vi "临界安全监督数据处理.vi"() -> ()   [LabVIEW 2020]
uses:
  <vilib>/Utility/miscctls.llb/LVAnnotationListTypeDef.ctl
  <vilib>/Analysis/6fits.llb/Curve Fitting Criteria.ctl
  <vilib>/Utility/miscctls.llb/LVRowAndColumnTypeDef.ctl
  <vilib>/Utility/inputDevices.llb/mouseAcquire.vi
  <vilib>/Analysis/NI_AALPro.lvlib
panel:
  in  "背景色":bool
  in  "临界途径选择":u16(ring)
  in  "表象周期标尺\n   手动调整":bool
  in  "Min+":bool
  in  "Min-":bool
  in  "Max+":bool
  in  "Max-":bool
  out "左选标时刻":timestamp
  out "总时长":dbl
  in  "保存表格":bool
  in  "添加记录":bool
  out "Table":string[][](table) caption="表格"
  out "Axis Info":T1 caption="轴信息"
  in  "曲线标尺":bool[](array[boolean])
  in  "曲线隐显":bool[](array[boolean])
  out "提示信息":string
  in  "开始计算":bool
  in  "重选文件":bool
  in  "退出程序":bool
  out "filepath":path caption="数据文件路径和名称"
  out "数据采集起止时间":string
  out "中间段数据个数":i32
  out "左选标位置":i32
  out "右选标位置":i32
  out "选段斜率":sgl[](array[numeric])
  out "通量平均值":sgl[](array[numeric])
  out "表象周期平均（秒）":sgl[](array[numeric])
  out "临界途径平均值":sgl[](array[numeric])
  out "【文件波形】":dbl[][](graph)
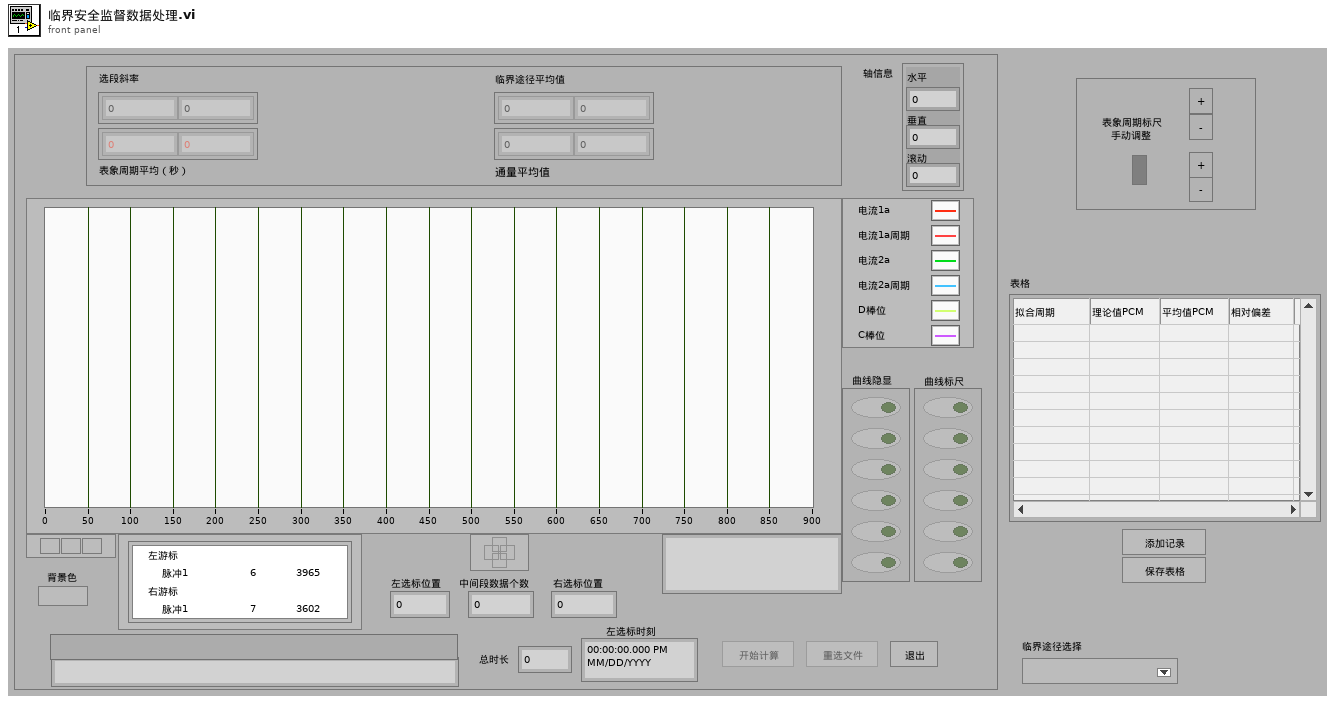
[diagram p1: front panel]
types:
  T1 = cluster{"Horizontal":i32, "Vertical":i32, "Scrolling":i32}
  T2 = enum8{"Enabled", "Disabled", "Disabled and Grayed Out"}
  T3 = typedef "LVAnnotationListTypeDef.ctl" = cluster{"Name":string, "Color":u32, "Style":u8, "Point Style":u8, "Name Visible":bool, "Allow Drag":bool, "Annotation Mode":u32, "Plot":i32, "Index":i32, "Position":cluster{"X":dbl, "Y":dbl}, "X Scale":u32, "Y Scale":u32, "Show Arrow":bool, "Lock Name":bool, "Plot Area":i32, "Label Offset":cluster{"X":dbl, "Y":dbl}}[]
  T4 = cluster{"Name":string, "Color":u32, "Style":u8, "Point Style":u8, "Name Visible":bool, "Allow Drag":bool, "Annotation Mode":u32, "Plot":i32, "Index":i32, "Position":cluster{"X":dbl, "Y":dbl}, "X Scale":u32, "Y Scale":u32, "Show Arrow":bool, "Lock Name":bool, "Plot Area":i32, "Label Offset":cluster{"X":dbl, "Y":dbl}}
  T5 = enum16{"open", "replace", "create", "open or create", "replace or create", "replace or create with confirmation"}
  T6 = typedef "LVRowAndColumnTypeDef.ctl" = cluster{"Row":i32, "Column":i32}
  T7 = cluster{"button 1":bool, "button 2":bool, "button 3":bool, "button 4":bool}
  T8 = typedef "LVCursorListTypeDef.ctl" = cluster{"Name":string, "Color":u32, "Style":u8, "Point Style":u8, "Name Visible":bool, "Allow Drag":bool, "Cursor Mode":u32, "Plot":i32, "Index":i32, "Position":cluster{"X":dbl, "Y":dbl}, "X Scale":u32, "Y Scale":u32, "Watch Plots":i32[], "Watch All Plots":bool, "Plot Area":i32, "Label Offset":cluster{"X":dbl, "Y":dbl}}[]
  T9 = cluster{"Name":string, "Color":u32, "Style":u8, "Point Style":u8, "Name Visible":bool, "Allow Drag":bool, "Cursor Mode":u32, "Plot":i32, "Index":i32, "Position":cluster{"X":dbl, "Y":dbl}, "X Scale":u32, "Y Scale":u32, "Watch Plots":i32[], "Watch All Plots":bool, "Plot Area":i32, "Label Offset":cluster{"X":dbl, "Y":dbl}}
  T10 = typedef "NI_AALPro.lvlib/Curve Fitting Criteria.ctl" = u16
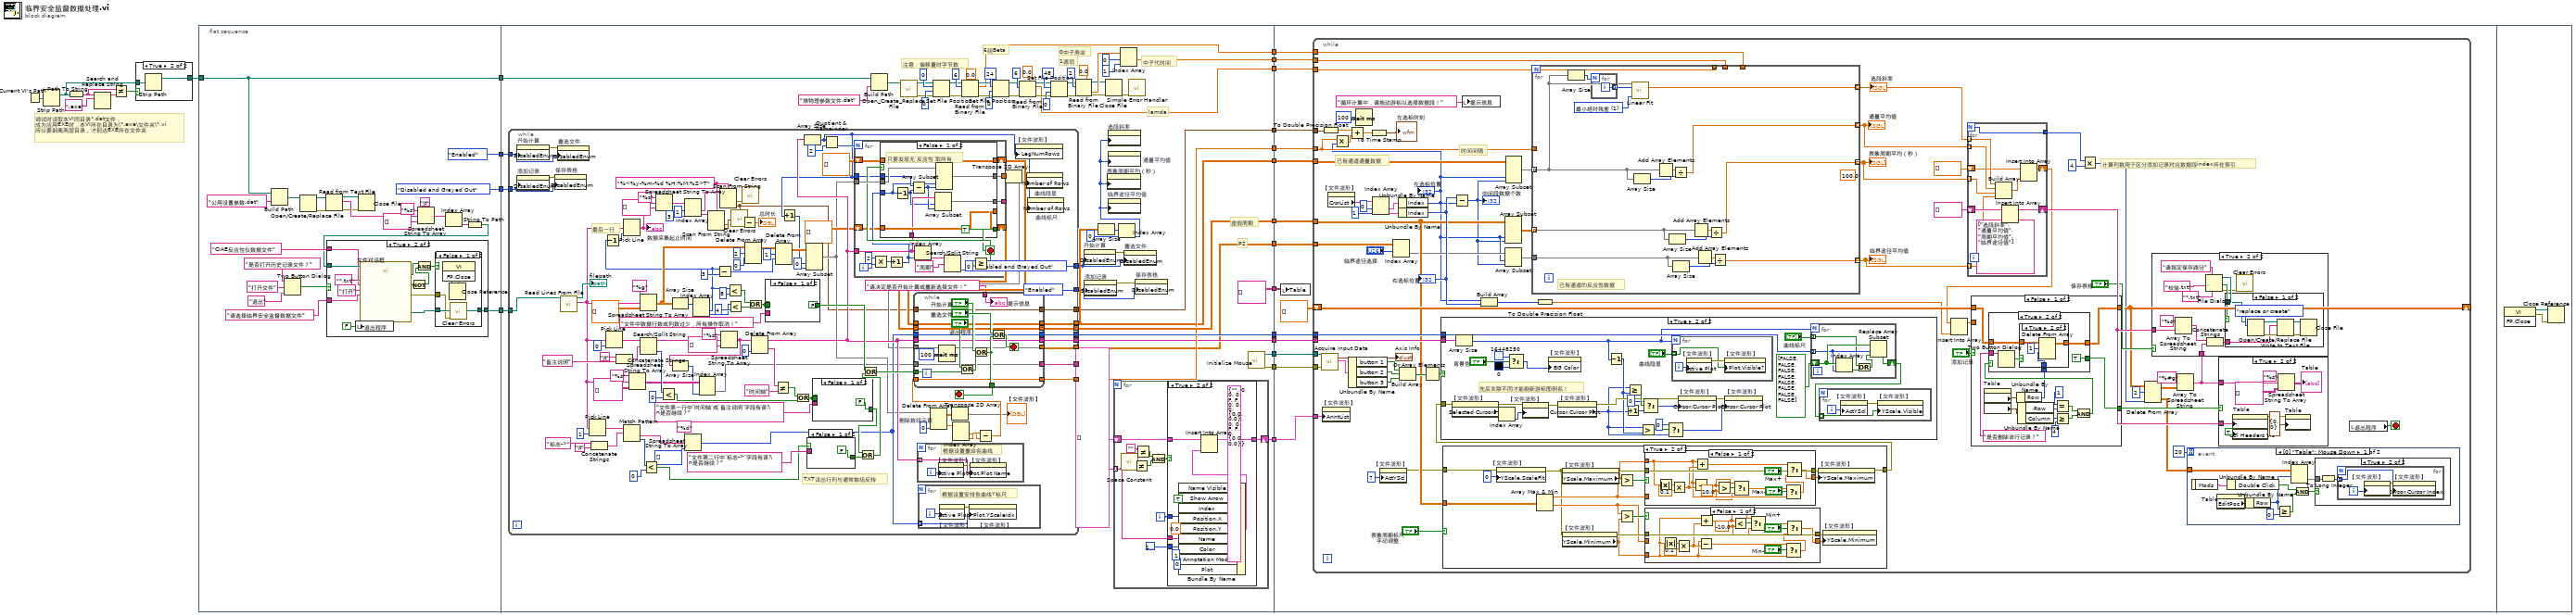
[diagram p0: block diagram]
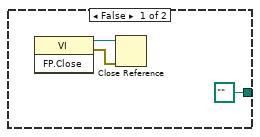
[diagram p3: hidden frame]
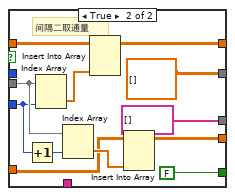
[diagram p6: hidden frame]
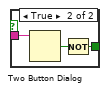
[diagram p7: hidden frame]
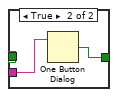
[diagram p8: hidden frame]
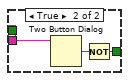
[diagram p9: hidden frame]
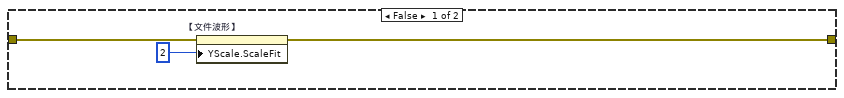
[diagram p10: hidden frame]
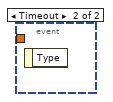
[diagram p14: hidden frame]
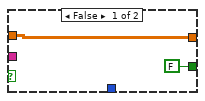
[diagram p18: hidden frame]
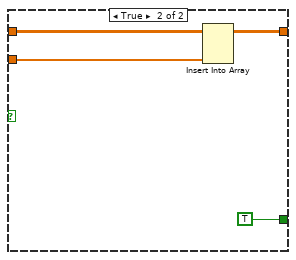
[diagram p20: hidden frame]
diagram:
  # "调试时读取本VI同目录*.dat文件，\n成为应用EXE时，本VI所在目录为\\*.exe\\文件夹\\*.vi\n所以要剥离两层目录，才到达EXE所在文件夹"
  n1 = Current VI's Path() -> (path=w4:path)
  n2 = Strip Path(path=w4) -> (stripped path=w9:path)  [unwired: 1 out]
  n3 = Path To String(path=w9) -> (string=w7:string)
  n4 = Search and Replace String(input string=w7, search string=".exe" ("搜索字符串")) -> (result string=w6:string)  [unwired: 6 in, 3 out]
  n5 = Not Equal?(x=w7, y=w6) -> (x != y?=w8:bool)
  n6 = case shown="True" w8 {
    tunnel: w9 -> [w26 w28]
    tunnel: [w26 w27] -> w3
    frame False {
    }
    frame True {
      n7 = Strip Path(path=w28) -> (stripped path=w27:path)  [unwired: 1 out]
    }
  }
  n8 = flat-sequence {
    tunnel: [T2."Enabled" ("禁用")] -> w13
    tunnel: [T2."Disabled and Grayed Out" ("禁用")] -> w12
    tunnel: w3 -> [w29]
    tunnel: [w29] -> w2
    tunnel: [w30] -> w1
    tunnel: [w96] -> w25
    tunnel: [w95] -> w24
    tunnel: [w94] -> w23
    tunnel: [w99] -> w22
    tunnel: [w98] -> w21
    tunnel: [w97] -> w20
    tunnel: [w90] -> w19
    tunnel: [w89] -> w18
    tunnel: [w88] -> w17
    tunnel: [w87] -> w16
    tunnel: [w85] -> w15
    tunnel: [string[][] [] ("添加的数组")] -> w14
    tunnel: w13 -> [w80]
    tunnel: w12 -> [w77]
    tunnel: [w76] -> w11
    tunnel: [w75] -> w10
    tunnel: w2 -> [w74]
    tunnel: w1 -> [w73]
    tunnel: w23 -> [w358]
    tunnel: w25 -> [w357]
    tunnel: w24 -> [w356]
    tunnel: w22 -> [w355]
    tunnel: w21 -> [w354]
    tunnel: w20 -> [w353]
    tunnel: w19 -> [w352]
    tunnel: w18 -> [w351]
    tunnel: w17 -> [w350]
    tunnel: w16 -> [w349]
    tunnel: w15 -> [w348]
    tunnel: w14 -> [w346]
    tunnel: w11 -> [w345]
    tunnel: w10 -> [w344]
    frame #0 {
      n9 = Build Path(base path=w29, name or relative path="公用设置参数.dat") -> (appended path=w36:path)
      n10 = Two Button Dialog(message="是否打开历史记录文件？", 1:"退出" ("message"), 2:"打开文件" ("message")) -> (T button?=w46:bool)
      n11 = Open/Create/Replace File(file path (use dialog)=w36) -> (refnum out=w39:refnum<file>, error out=w40:errorcluster)  [unwired: 5 in, 1 out]
      n12 = Read from Text File(file (use dialog)=w39, error in=w40) -> (refnum out=w38:refnum<file>, text=w44:string, error out=w37:errorcluster)  [unwired: 1 in, 2 out]
      n13 = Close File(refnum=w38, error in=w37) -> ()  [unwired: 2 out]
      n14 = Spreadsheet String To Array(delimiter (Tab)="\t", format string="%s", spreadsheet string=w44, array type (2D Dbl)=string[] [] ("添加的数组")) -> (array=w45:string[])
      n15 = Index Array(array=w45) -> (element=w34:string)  [unwired: 1 in]
      n16 = String To Path(string=w34) -> (path=w47:path)
      n17 = case shown="True" w46 {
        tunnel: w47 -> [_ w67]
        tunnel: "请选择临界安全监督数据文件" ("prompt") -> [_ w63]
        tunnel: "CIAE反应性仪数据文件" ("pattern label") -> [_ w62]
        tunnel: [path "" ("selected path") w60] -> w30
        frame False {
          n18 = invoke class="VI" method="FP.Close"() -> (reference out=w53:refnum<vi>, error out=w52:errorcluster)  [unwired: 3 in, 1 out]
          n19 = Close Reference(reference=w53, error in (no error)=w52) -> ()  [unwired: 1 out]
        }
        frame True {
          n20 = local write "退出程序"(FALSE ("退出程序")) -> ()
          n21 = call "文件对话框"("start path"=w67, "prompt"=w63, "button label"="打开", "pattern (all files)"="*.txt", "pattern label"=w62) -> ("selected path"=w61:path, "exists"=w58:bool, "cancelled"=w59:bool, "error out"=w55:errorcluster)  [unwired: 7 in]
          n22 = Not(x=w59) -> (.not. x?=w57:bool)
          n23 = And(x=w58, y=w57) -> (x .and. y?=w56:bool)
          n24 = case shown="False" w56 {
            tunnel: w61 -> [w71 w72]
            tunnel: [w71 w72] -> w60
            tunnel: w55 -> [w68 _]
            frame False {
              n25 = invoke class="VI" method="FP.Close"() -> (reference out=w69:refnum<vi>, error out=w70:errorcluster)  [unwired: 3 in, 1 out]
              n26 = Close Reference(reference=w69, error in (no error)=w70) -> ()  [unwired: 1 out]
              n27 = call <vilib>:"Clear Errors.vi"("error in (no error)"=w68) -> ()  [unwired: 5 in, 2 out]
            }
            frame True {
            }
          }
        }
      }
    }
    frame #1 {
      # "虚假周期"
      # "P2"
      # "注意：偏移量时字节数"
      # "0中子寿命"
      # "1源项"
      # "6组Beta"
      # "中子代时间"
      # "lamda"
      n28 = while {
        tunnel: [w212] -> w96
        tunnel: [w260] -> w90
        tunnel: [w209] -> w89
        tunnel: [w210] -> w94
        tunnel: [w198] -> w95
        tunnel: [w181] -> w86
        tunnel: [T2."Disabled and Grayed Out" ("禁用")] -> w81
        tunnel: w80 -> [w177]
        tunnel: [T2."Enabled" ("禁用")] -> w78
        tunnel: w77 -> [w174]
        tunnel: [w170] -> w76
        tunnel: [w155] -> w75
        tunnel: w73 -> [w154]
        stop <- w266 stop-if-true
        w161 = "%<%y-%m-%d %H:%M:%S>T" ("格式字符串")
        # "TXT读出行列与通常数组反转"
        # "最后一行"
        n29 = property on="开始计算" class="Bool"("DisabledEnum"=w177) -> (error out=w178:errorcluster)  [unwired: 2 in, 1 out]
        n30 = property on="添加记录" class="Bool"("DisabledEnum"=w174) -> (error out=w175:errorcluster)  [unwired: 2 in, 1 out]
        n31 = property on="保存表格" class="Bool"(error in=w175, "DisabledEnum"=w174) -> ()  [unwired: 1 in, 2 out]
        n32 = property on="重选文件" class="Bool"(error in=w178, "DisabledEnum"=w177) -> ()  [unwired: 1 in, 2 out]
        n33 = call <vilib>:"Read Lines From File.vi"("file path (dialog if empty)"=w154) -> ("new file path (Not A Path if cancelled)"=→"filepath":path, "line string"=w186:string)  [unwired: 5 in, 2 out]
        n34 = Pick Line(multi-line string=w186, line index=1 ("行索引")) -> (output string=w239:string)  [unwired: 1 in]
        n35 = Concatenate Strings("标志->" ("搜索字符串/字符(-)"), "\t") -> (w236:string)
        n36 = Pick Line(multi-line string=w186, line index=0 ("行索引")) -> (output string=w258:string)  [unwired: 1 in]
        n37 = Concatenate Strings("\t", "备注说明" ("搜索字符串/字符(-)")) -> (w219:string)
        n38 = Match Pattern(string=w239, regular expression=w236) -> (after substring=w233:string, offset past match=w227:i32)  [unwired: 1 in, 2 out]
        n39 = Spreadsheet String To Array ("电子表格字符串至数组转换")(format string="%s" ("format (%.3f)"), spreadsheet string=w186, array type (2D Dbl)=string[][] [] ("添加的数组")) -> (array=w185:string[][])  [unwired: 1 in]
        n40 = Spreadsheet String To Array ("电子表格字符串至数组转换")(format string="%g" ("format (%.3f)"), spreadsheet string=w186, array type (2D Dbl)=dbl[][] [] ("type (empty)")) -> (array=w221:dbl[][])  [unwired: 1 in]
        n41 = Search/Split String(string=w258, search string/char (-)=w219) -> (substring before match=w257:string, offset of match=w256:i32)  [unwired: 1 in, 1 out]
        n42 = Less?(x=w227, y=0) -> (x < y?=w226:bool)
        n43 = Less?(x=w256, y=0) -> (x < y?=w253:bool)
        n44 = Array Size(array=w221) -> (size(s)=w267:i32[])
        n45 = Spreadsheet String To Array ("电子表格字符串至数组转换")(format string="%d" ("format (%.3f)"), spreadsheet string=w233, array type (2D Dbl)=i32[] [] ("添加的数组")) -> (array=w207:i32[])  [unwired: 1 in]
        n46 = Index Array(array=w267) -> (element #1=w171:i32, element #2=w247:i32)  [unwired: 2 in]
        n47 = Decrement(x=w171) -> (x-1=w172:i32)
        n48 = Pick Line(multi-line string=w186, line index=w172) -> (output string=w169:string)  [unwired: 1 in]
        "数据采集起止时间" <- w169
        n49 = Spreadsheet String To Array(format string="%s" ("格式字符串"), spreadsheet string=w169, array type (2D Dbl)=string[] [] ("添加的数组")) -> (array=w166:string[])  [unwired: 1 in]
        n50 = Index Array(array=w166, index #1=1 ("索引"), index #2=3 ("索引")) -> (element #1=w163:string, element #2=w162:string)
        n51 = Scan From String(format string=w161, input string=w162) -> (error out=w156:errorcluster, output 1=w160:timestamp)  [unwired: 3 in, 2 out]
        n52 = Subtract(x=w171, y=3) -> (x-y=w216:i32)
        n53 = Scan From String(format string=w161, input string=w163) -> (error out=w157:errorcluster, output 1=w159:timestamp)  [unwired: 3 in, 2 out]
        n54 = Spreadsheet String To Array ("电子表格字符串至数组转换")(format string="%s" ("format (%.3f)"), spreadsheet string=w257, array type (2D Dbl)=string[] [] ("添加的数组")) -> (array=w184:string[])  [unwired: 1 in]
        n55 = Array Size(array=w184) -> (size(s)=w183:i32)
        n56 = Index Array(array=w185, index (col)=w183) -> (element=w182:string[])  [unwired: 1 in]
        n57 = Less?(x=w171, y=8) -> (x < y?=w245:bool)
        n58 = Less?(x=w247, y=4) -> (x < y?=w244:bool)
        n59 = call <vilib>:"Clear Errors.vi"("error in (no error)"=w156) -> ()  [unwired: 5 in, 2 out]
        n60 = Subtract(x=w160, y=w159) -> (x-y=→"总时长":dbl)
        n61 = call <vilib>:"Clear Errors.vi"("error in (no error)"=w157) -> ()  [unwired: 5 in, 2 out]
        n62 = Delete From Array(array=w221, length=2 ("长度"), index (row)=0 ("索引")) -> (array with subset deleted=w220:dbl[][])  [unwired: 1 in, 1 out]
        n63 = Or(x=w245, y=w244) -> (x .or. y?=w246:bool)
        n64 = Delete From Array(array=w184, index=0 ("索引")) -> (deleted portion=w194:string, array with subset deleted=w208:string[])  [unwired: 1 in]
        n65 = case shown="False" w246 {
          tunnel: w246 -> [_ _]
          tunnel: [FALSE w321] -> w241
          tunnel: "文件中数据行数或列数过少，所有操作取消！" ("y") -> [_ w322]
          frame False {
          }
          frame True {
            n66 = One Button Dialog(message=w322) -> (true=w321:bool)  [unwired: 1 in]
          }
        }
        n67 = Not Equal?(x=w194, y="时间轴") -> (x != y?=w252:bool)
        n68 = Delete From Array(array=w220, length=1 ("长度"), index (row)=w216) -> (array with subset deleted=w193:dbl[][])  [unwired: 1 in, 1 out]
        n69 = Or(x=w252, y=w253) -> (x .or. y?=w251:bool)
        n70 = Array Size(array=w208) -> (size(s)=w189:i32)
        n71 = Increment(x=w189) -> (x+1=w190:i32)
        n72 = Array Subset(array=w193, index (col)=0 ("索引"), length (col)=w190) -> (w192:dbl[][])  [unwired: 2 in]
        n73 = case shown="False" w226 {
          tunnel: "文件第二行中‘标志->’字段有误!\n是否继续？" ("y") -> [_ w319]
          tunnel: [FALSE w317] -> w231
          frame False {
          }
          frame True {
            n74 = Two Button Dialog(message=w319) -> (T button?=w318:bool)  [unwired: 2 in]
            n75 = Not(x=w318) -> (.not. x?=w317:bool)
          }
        }
        n76 = case shown="False" w251 {
          tunnel: w251 -> [_ _]
          tunnel: "文件第一行中‘时间轴’或‘备注说明’字段有误!\n是否继续？" ("y") -> [_ w326]
          tunnel: [FALSE w324] -> w230
          frame False {
          }
          frame True {
            n77 = Two Button Dialog(message=w326) -> (T button?=w325:bool)  [unwired: 2 in]
            n78 = Not(x=w325) -> (.not. x?=w324:bool)
          }
        }
        n79 = Quotient & Remainder(x=w189, y=2) -> (floor(x/y)=w213:i32)  [unwired: 1 out]
        n80 = for {
          N: w213 -> [_]
          tunnel: w192 -> [w286]
          tunnel: w208 -> [w275]
          shift-right: [w284] -> w197
          shift-left: dbl[][] [] ("type (empty)") -> [w285]
          tunnel: w189 -> [w280]
          tunnel: [w279] -> w211
          shift-right: [w276] -> w203
          shift-left: dbl[][] [] ("type (empty)") -> [w277]
          tunnel: [w274] -> _
          i -> [w292]
          stop <- w281 stop-if-true
          n81 = Multiply(x=2, y=w292) -> (x*y=w278:i32)
          n82 = Increment(x=w278) -> (x+1=w282:i32)
          n83 = Index Array(array=w275, index=w282) -> (element=w290:string)
          n84 = Search/Split String(string=w290, search string/char (-)="周期" ("搜索字符串/字符(-)")) -> (offset of match=w288:i32)  [unwired: 1 in, 2 out]
          n85 = Greater Or Equal?(x=w288, y=0) -> (x >= y?=w283:bool)
          n86 = case shown="False" w283 {
            tunnel: w286 -> [w301 w310]
            tunnel: w285 -> [w303 w315]
            tunnel: [w303 w313] -> w284
            tunnel: w282 -> [w296 w305]
            tunnel: [TRUE FALSE] -> w281
            tunnel: w280 -> [w300 _]
            tunnel: [w299 dbl[][] [] ("type (empty)")] -> w279
            tunnel: w277 -> [w298 w308]
            tunnel: [w298 w307] -> w276
            tunnel: w275 -> [w297 _]
            tunnel: [w294 string[] []] -> w274
            frame False {
              # "只要发现无‘反应性’取所有"
              n87 = Decrement(x=w296) -> (x-1=w293:i32)
              n88 = Subtract(x=w300, y=w293) -> (x-y=w295:i32)
              n89 = Array Subset(array=w297, index=w293, length=w295) -> (w294:string[])
              n90 = Array Subset(array=w301, index (col)=w296, length (col)=w295) -> (w299:dbl[][])  [unwired: 2 in]
            }
            frame True {
              # "间隔二取通量"
              n91 = Increment(x=w305) -> (x+1=w306:i32)
              n92 = Index Array(array=w310, index (col)=w305) -> (element=w314:dbl[])  [unwired: 1 in]
              n93 = Index Array(array=w310, index (col)=w306) -> (element=w309:dbl[])  [unwired: 1 in]
              n94 = Insert Into Array(array=w315, new element=w314) -> (w313:dbl[][])  [unwired: 2 in]
              n95 = Insert Into Array(array=w308, new element=w309) -> (w307:dbl[][])  [unwired: 2 in]
            }
          }
        }
        n96 = Or(x=w230, y=w231) -> (x .or. y?=w229:bool)
        n97 = Or(x=w241, y=w229) -> (x .or. y?=w242:bool)
        n98 = for {
          tunnel: w208 -> [w272] mode=indexing
          i -> [w273]
          # "根据设置重命名曲线"
          n99 = property on="【文件波形】" class="WFGraph (strict)"("Active Plot"=w273) -> (error out=w271:errorcluster)  [unwired: 2 in, 1 out]
          n100 = property on="【文件波形】" class="WFGraph (strict)"(error in=w271, "Plot.Plot Name"=w272) -> ()  [unwired: 1 in, 2 out]
        }
        n101 = for {
          tunnel: w207 -> [w268] mode=indexing
          i -> [w270]
          # "根据设置安排各曲线Y标尺"
          n102 = property on="【文件波形】" class="WFGraph (strict)"("Active Plot"=w270) -> (error out=w269:errorcluster)  [unwired: 2 in, 1 out]
          n103 = property on="【文件波形】" class="WFGraph (strict)"(error in=w269, "Plot.YScaleIdx"=w268) -> ()  [unwired: 1 in, 2 out]
        }
        n104 = Delete From Array "删除数组元素"(array=w192, index (col)=0 ("禁用的索引 (列)")) -> (deleted portion=w202:dbl[], array with subset deleted=w206:dbl[][])  [unwired: 2 in]
        n105 = Transpose 2D Array(2D array=w206) -> (transposed array=→"【文件波形】":dbl[][])
        n106 = Index Array(array=w202) -> (element #1=w200:dbl, element #2=w201:dbl)  [unwired: 2 in]
        n107 = Subtract(x=w201, y=w200) -> (x-y=w199:dbl)
        n108 = Transpose 2D Array(2D array=w211) -> (transposed array=w180:dbl[][])
        n109 = while {
          tunnel: [w334] -> w212
          tunnel: [w332] -> w260
          tunnel: w203 -> [w334]
          tunnel: w208 -> [w332]
          tunnel: [w341] -> w266
          tunnel: w242 -> [w337]
          tunnel: w197 -> [w335]
          tunnel: [w335] -> w210
          tunnel: w207 -> [w333]
          tunnel: [w333] -> w209
          tunnel: w199 -> [w331]
          tunnel: [w331] -> w198
          tunnel: "请决定是否开始计算或重新选择文件！" ("提示信息") -> [w330]
          tunnel: [w329] -> w181
          tunnel: w182 -> [w329]
          tunnel: [w328] -> w155
          tunnel: w180 -> [w328]
          tunnel: [w327] -> w170
          tunnel: w159 -> [w327]
          stop <- w340 stop-if-true
          n110 = Wait (ms)(milliseconds to wait=u32 100 ("等待时间（毫秒）")) -> ()  [unwired: 1 out]
          n111 = Or(x="退出程序", y=w337) -> (x .or. y?=w338:bool)
          n112 = Or(x="开始计算", y=w338) -> (x .or. y?=w341:bool)
          n113 = Or(x="重选文件", y=w341) -> (x .or. y?=w340:bool)
          "提示信息" <- w330
        }
        n114 = property on="【文件波形】" class="WFGraph (strict)"("LegNumRows"=w189) -> ()  [unwired: 2 in, 2 out]
        n115 = property on="曲线隐显" class="Arr (strict)"("Number of Rows"=w189) -> ()  [unwired: 2 in, 2 out]
        n116 = property on="曲线标尺" class="Arr (strict)"("Number of Rows"=w189) -> ()  [unwired: 2 in, 2 out]
      }
      n117 = Build Path(base path=w74, name or relative path="堆物理参数文件.dat" ("string")) -> (appended path=w115:path)
      n118 = call <vilib>:"Open_Create_Replace File.vi"("file path"=w115) -> ("error out"=w100:errorcluster, "refnum"=w101:refnum<file>)  [unwired: 7 in, 2 out]
      n119 = Set File Position(offset (in bytes) (0)=0, refnum=w101, from (0:start)=0, error in=w100) -> (refnum out=w112:refnum<file>, error out=w111:errorcluster)
      n120 = Read from Binary File(5:sgl 0.0, 8:w111, 10:6, 11:w112) -> (0:w107:errorcluster, 2:w99:sgl[], 3:w108:refnum<file>)  [unwired: 2 in, 1 out]
      n121 = Set File Position(offset (in bytes) (0)=24, refnum=w108, from (0:start)=0, error in=w107) -> (refnum out=w110:refnum<file>, error out=w109:errorcluster)
      n122 = Read from Binary File(5:sgl 0.0, 8:w109, 10:6, 11:w110) -> (0:w105:errorcluster, 2:w98:sgl[], 3:w106:refnum<file>)  [unwired: 2 in, 1 out]
      n123 = Set File Position(offset (in bytes) (0)=48, refnum=w106, from (0:start)=0, error in=w105) -> (refnum out=w114:refnum<file>, error out=w113:errorcluster)
      n124 = Read from Binary File(5:sgl 0.0, 8:w113, 10:2, 11:w114) -> (0:w103:errorcluster, 2:w123:sgl[], 3:w104:refnum<file>)  [unwired: 2 in, 1 out]
      n125 = property on="开始计算" class="Bool"("DisabledEnum"=w81) -> (error out=w82:errorcluster)  [unwired: 2 in, 1 out]
      n126 = property on="添加记录" class="Bool"("DisabledEnum"=w78) -> (error out=w79:errorcluster)  [unwired: 2 in, 1 out]
      n127 = Array Size(array=w94) -> (size(s)=w93:i32[])
      n128 = Close File(refnum=w104, error in=w103) -> (error out=w102:errorcluster)  [unwired: 1 out]
      n129 = for {
        tunnel: w86 -> [w136] mode=indexing
        shift-right: [w138] -> w85
        shift-left: T3 [] ("注释列表") -> [w139]
        i -> [w140]
        n130 = call <vilib>:"Space Constant.vi"() -> ("String"=w141:string)
        n131 = Not Equal?(x=w141, y=w136) -> (x != y?=w134:bool)
        n132 = Not Equal?(x="", y=w136) -> (x != y?=w135:bool)
        n133 = And(x=w135, y=w134) -> (x .and. y?=w133:bool)
        n134 = case shown="True" w133 {
          tunnel: w136 -> [_ w148]
          tunnel: w140 -> [_ w150]
          tunnel: w139 -> [w142 w153]
          tunnel: [w142 w152] -> w138
          tunnel: u32 16777228 -> [_ w145]
          frame False {
          }
          frame True {
            w151 = TRUE ("Show Arrow")
            n135 = Bundle By Name(cluster=T4 {"Name"="", "Color"=0, "Style"=0, "Point Style"=0, "Name Visible"=FALSE, "Allow Drag"=FALSE, "Annotation Mode"=0, "Plot"=0, "Index"=0, "Position"={"X"=0.0, "Y"=0.0}, "X Scale"=0, "Y Scale"=0, "Show Arrow"=FALSE, "Lock Name"=FALSE, "Plot Area"=0, "Label Offset"={"X"=0.0, "Y"=0.0}} ("元素"), "Name Visible"=w151, "Show Arrow"=w151, "Index"=w150, "Position.X"=w150, "Position.Y"=0.0 ("Y"), "Name"=w148, "Color"=w145, "Annotation Mode"=u32 1, "Plot"=0) -> (w149:T4)
            n136 = Insert Into Array(array=w153, new element=w149) -> (w152:T3)  [unwired: 1 in]
          }
        }
      }
      n137 = Index Array(array=w93, index=0 ("索引")) -> (element=w92:i32)
      n138 = property on="表象周期平均（秒）" class="Arr (strict)"("Number of Columns"=w92) -> ()  [unwired: 2 in, 2 out]
      n139 = property on="选段斜率" class="Arr (strict)"("Number of Columns"=w92) -> ()  [unwired: 2 in, 2 out]
      n140 = property on="通量平均值" class="Arr (strict)"("Number of Columns"=w92) -> ()  [unwired: 2 in, 2 out]
      n141 = property on="临界途径平均值" class="Arr (strict)"("Number of Columns"=w92) -> ()  [unwired: 2 in, 2 out]
      n142 = Index Array(array=w123, index #1=0, index #2=1) -> (element #1=w97:sgl)  [unwired: 1 out]
      n143 = property on="重选文件" class="Bool"(error in=w82, "DisabledEnum"=w81) -> ()  [unwired: 1 in, 2 out]
      n144 = call <vilib>:"Simple Error Handler.vi"("error in (no error)"=w102) -> ()  [unwired: 4 in, 5 out]
      n145 = property on="保存表格" class="Bool"(error in=w79, "DisabledEnum"=w78) -> ()  [unwired: 1 in, 2 out]
      n146 = call <vilib>:"Initialize Mouse.vi"() -> ("error out"=w87:errorcluster, "device ID"=w88:refnum<k1>)  [unwired: 1 in, 9 out]
    }
    frame #2 {
      n147 = local write "Table"(w346) -> ()
      n148 = while {
        tunnel: w358 -> [w422]
        tunnel: w357 -> [w368]
        tunnel: w356 -> [w370]
        tunnel: w355 -> [w420]
        tunnel: w354 -> [w419]
        tunnel: w353 -> [w418]
        tunnel: w352 -> [w413]
        tunnel: w351 -> [w412]
        tunnel: w350 -> [w409]
        tunnel: w349 -> [w408]
        tunnel: w348 -> [w402]
        shift-right: [w386] -> _
        shift-left: dbl[][] [] ("type (empty)") -> [w396]
        tunnel: w345 -> [w375]
        tunnel: w344 -> [w364]
        stop <- w415 stop-if-true
        # "时间间隔"
        # "计算列数用于区分添加记录对应数据段index所在索引"
        # "已有通道通量数据"
        n149 = call-poly <vilib>:"Acquire Input Data.vi"("device ID"=w409, "error in (no error)"=w408) -> ("axis info"=→"Axis Info":T1, "button info"=w410:T7)  [unwired: 1 in, 15 out]
        n150 = property on="【文件波形】" class="WFGraph (strict)"("AnntList"=w402) -> ()  [unwired: 2 in, 2 out]
        n151 = To Double Precision Float(number=w375) -> (double precision float=w374:dbl)
        n152 = property on="【文件波形】" class="WFGraph (strict)"() -> ("CrsrList"=w423:T8)  [unwired: 2 in, 2 out]
        n153 = Unbundle By Name(w410) -> ("button 1"=w407:bool, "button 2"=w406:bool, "button 3"=w405:bool)
        n154 = Wait (ms)(milliseconds to wait=u32 100 ("等待时间（毫秒）")) -> ()  [unwired: 1 out]
        n155 = Index Array(array=w423, index #1=0 ("index"), index #2=1 ("index")) -> (element #1=w425:T9, element #2=w427:T9)
        n156 = property on="【文件波形】" class="WFGraph (strict)"("ActYScl"=7 ("活动Y标尺")) -> (error out=w366:errorcluster)  [unwired: 2 in, 1 out]
        n157 = Index Array(array=w364, index (row)="临界途径选择") -> (element=w362:dbl[])  [unwired: 1 in]
        n158 = Unbundle By Name(w425) -> ("Index"=w361:i32)
        "左选标位置" <- w361
        n159 = Multiply(x=w370, y=w361) -> (x*y=w371:dbl)
        n160 = Add(x=w374, y=w371) -> (x+y=w373:dbl)
        n161 = To Time Stamp(1:w373) -> (0:→"左选标时刻":timestamp)
        n162 = Unbundle By Name(w427) -> ("Index"=w380:i32)
        "右选标位置" <- w380
        n163 = Build Array(w407, w406, w405) -> (w404:bool[])
        n164 = Or Array Elements(Boolean array=w404) -> (logical OR=w403:bool)
        n165 = case shown="True" "表象周期标尺\n   手动调整" {
          tunnel: w368 -> [_ w441]
          tunnel: w366 -> [w429 w432]
          tunnel: [w428 w431] -> w365
          frame False {
            n166 = property on="【文件波形】" class="WFGraph (strict)"(error in=w429, "YScale.ScaleFit"=u8 2 ("Y标尺.标尺调节")) -> (error out=w428:errorcluster)  [unwired: 1 in, 1 out]
          }
          frame True {
            n167 = property on="【文件波形】" class="WFGraph (strict)"(error in=w432, "YScale.ScaleFit"=u8 0 ("Y标尺.标尺调节")) -> (error out=w434:errorcluster)  [unwired: 1 in, 1 out]
            n168 = Array Max & Min(array=w441) -> (max value=w443:dbl, min value=w444:dbl)  [unwired: 2 out]
            n169 = property on="【文件波形】" class="WFGraph (strict)"(error in=w434) -> (error out=w447:errorcluster, "YScale.Maximum"=w436:dbl)  [unwired: 1 in, 1 out]
            n170 = property on="【文件波形】" class="WFGraph (strict)"(error in=w434) -> (error out=w446:errorcluster, "YScale.Minimum"=w435:dbl)  [unwired: 1 in, 1 out]
            n171 = Greater?(x=w436, y=w443) -> (0:w442:bool)
            n172 = Greater?(x=w444, y=w435) -> (0:w445:bool)
            n173 = case shown="False" w442 {
              tunnel: w443 -> [_ w463]
              tunnel: w447 -> [w461 w462]
              tunnel: [w453 w463] -> w440
              tunnel: [w461 w462] -> w439
              tunnel: w436 -> [w452 _]
              frame False {
                w449 = 10.0 ("y")
                n174 = Absolute Value(x=w452) -> (abs(x)=w457:dbl)
                n175 = Multiply(x=w457, y=0.1) -> (x*y=w459:dbl)
                n176 = Subtract(x=w452, y=w459) -> (x-y=w450:dbl)
                n177 = Add(x=w452, y=w459) -> (x+y=w460:dbl)
                n178 = Greater?(x=w450, y=w449) -> (0:w451:bool)
                n179 = Select(t=w450, s=w451, f=w449) -> (s? t:f=w448:dbl)
                n180 = Select(t=w448, s="Max-", f=w452) -> (s? t:f=w454:dbl)
                n181 = Select(t=w460, s="Max+", f=w454) -> (s? t:f=w453:dbl)
              }
              frame True {
              }
            }
            n182 = case shown="False" w445 {
              tunnel: w444 -> [_ w479]
              tunnel: w446 -> [w477 w478]
              tunnel: [w473 w479] -> w438
              tunnel: [w477 w478] -> w437
              tunnel: w435 -> [w469 _]
              frame False {
                w467 = -10.0 ("y")
                n183 = Absolute Value(x=w469) -> (abs(x)=w472:dbl)
                n184 = Multiply(x=w472, y=0.1) -> (x*y=w470:dbl)
                n185 = Subtract(x=w469, y=w470) -> (x-y=w468:dbl)
                n186 = Add(x=w469, y=w470) -> (x+y=w464:dbl)
                n187 = Less?(x=w464, y=w467) -> (x < y?=w466:bool)
                n188 = Select(t=w464, s=w466, f=w467) -> (s? t:f=w465:dbl)
                n189 = Select(t=w468, s="Min-", f=w469) -> (s? t:f=w474:dbl)
                n190 = Select(t=w465, s="Min+", f=w474) -> (s? t:f=w473:dbl)
              }
              frame True {
              }
            }
            n191 = property on="【文件波形】" class="WFGraph (strict)"(error in=w439, "YScale.Maximum"=w440) -> (error out=w431:errorcluster)  [unwired: 1 in, 1 out]
            n192 = property on="【文件波形】" class="WFGraph (strict)"(error in=w437, "YScale.Minimum"=w438) -> ()  [unwired: 1 in, 2 out]
          }
        }
        n193 = case shown="True" w403 {
          tunnel: w413 -> [_ w580]
          tunnel: w412 -> [_ w579]
          tunnel: w365 -> [_ w566]
          frame False {
          }
          frame True {
            # "先后关联不同才能刷新游标图例名！"
            n194 = property on="【文件波形】" class="WFGraph (strict)"(error in=w566) -> (error out=w586:errorcluster, "Selected Cursors"=w588:u32[])  [unwired: 1 in, 1 out]
            n195 = Array Size(array=w580) -> (size(s)=w575:i32)
            n196 = Index Array(array=w588) -> (element=w587:u32)  [unwired: 1 in]
            n197 = Select(t=u32 16448250, s="背景色", f=u32 0) -> (s? t:f=w564:u32)
            n198 = property on="【文件波形】" class="WFGraph (strict)"(error in=w586, "Active Cursor"=w587) -> (error out=w585:errorcluster)  [unwired: 1 in, 1 out]
            n199 = property on="【文件波形】" class="WFGraph (strict)"("BG Color"=w564) -> ()  [unwired: 2 in, 2 out]
            n200 = property on="【文件波形】" class="WFGraph (strict)"(error in=w585) -> (error out=w582:errorcluster, "Cursor.Cursor Plot"=w568:i32)  [unwired: 1 in, 1 out]
            n201 = Decrement(x=w575) -> (x-1=w570:i32)
            n202 = Increment(x=w568) -> (x+1=w572:i32)
            n203 = Greater Or Equal?(x=w568, y=w570) -> (x >= y?=w584:bool)
            n204 = Greater?(x=w568, y=w570) -> (0:w571:bool)
            n205 = Select(t=0, s=w584, f=w572) -> (s? t:f=w574:i32)
            n206 = Select(t=0, s=w571, f=w568) -> (s? t:f=w569:i32)
            n207 = for {
              N: w575 -> [_]
              tunnel: "曲线隐显" -> [w592] mode=indexing
              i -> [w593]
              n208 = property on="【文件波形】" class="WFGraph (strict)"("Active Plot"=w593) -> (error out=w594:errorcluster)  [unwired: 2 in, 1 out]
              n209 = property on="【文件波形】" class="WFGraph (strict)"(error in=w594, "Plot.Visible?"=w592) -> ()  [unwired: 1 in, 2 out]
            }
            n210 = property on="【文件波形】" class="WFGraph (strict)"(error in=w582, "Cursor.Cursor Plot"=w574) -> (error out=w583:errorcluster)  [unwired: 1 in, 1 out]
            n211 = property on="【文件波形】" class="WFGraph (strict)"(error in=w583, "Cursor.Cursor Plot"=w569) -> ()  [unwired: 1 in, 2 out]
            n212 = for {
              N: w575 -> [_]
              tunnel: w579 -> [w599] mode=indexing
              tunnel: "曲线标尺" -> [w597] mode=indexing
              shift-right: [w595] -> w576
              shift-left: bool[] [FALSE, FALSE, FALSE, FALSE, FALSE, FALSE, FALSE, FALSE] ("曲线标尺") -> [w600]
              n213 = Index Array(array=w600, index=w599) -> (element=w598:bool)
              n214 = Or(x=w597, y=w598) -> (x .or. y?=w596:bool)
              n215 = Replace Array Subset(array=w600, new element=w596, index=w599) -> (w595:bool[])
            }
            n216 = for {
              tunnel: w576 -> [w590] mode=indexing
              i -> [w591]
              n217 = property on="【文件波形】" class="WFGraph (strict)"("ActYScl"=w591) -> (error out=w589:errorcluster)  [unwired: 2 in, 1 out]
              n218 = property on="【文件波形】" class="WFGraph (strict)"(error in=w589, "YScale.Visible"=w590) -> ()  [unwired: 1 in, 2 out]
            }
          }
        }
        n219 = Subtract(x=w380, y=w361) -> (x-y=w360:i32)
        "中间段数据个数" <- w360
        n220 = local write "提示信息"("循环计算中，请拖动游标以选择数据段！" ("提示信息")) -> ()
        n221 = Build Array(w361, w380) -> (w379:i32[])
        n222 = Array Subset(array=w368, index (col)=w361, length (col)=w360) -> (w417:dbl[][])  [unwired: 2 in]
        n223 = Array Subset(array=w362, index=w361, length=w360) -> (w359:dbl[])
        n224 = Array Subset(array=w422, index (col)=w361, length (col)=w360) -> (w421:dbl[][])  [unwired: 2 in]
        n225 = for {
          tunnel: w421 -> [w604] mode=indexing
          tunnel: w418 -> [_]
          tunnel: w420 -> [_]
          tunnel: w419 -> [_]
          tunnel: w417 -> [w616] mode=indexing
          tunnel: [w612] -> w400 mode=indexing
          tunnel: [w608] -> w398 mode=indexing
          tunnel: [w605] -> w401 mode=indexing
          tunnel: [w601] -> w399 mode=indexing
          tunnel: w370 -> [_]
          tunnel: w359 -> [w609]
          w602 = T10 1 items=["最小二乘", "最小绝对残差", "Bisquare"] ("method")
          (unwired) sgl 100.0 ("y")
          # "已有通道的反应性数据"
          n226 = Array Size(array=w604) -> (size(s)=w613:i32)
          n227 = for {
            N: w613 -> [_]
            tunnel: [w617] -> w603 mode=indexing
            i -> [w617]
          }
          n228 = call <vilib>:"Linear Fit.vi"("Y"=w604, "X"=w603, "method"=w602) -> ("slope"=w601:dbl)  [unwired: 8 in, 4 out]
          n229 = Array Size(array=w604) -> (size(s)=w606:i32)
          n230 = Add Array Elements(numeric array=w604) -> (sum=w607:dbl)
          n231 = Array Size(array=w616) -> (size(s)=w614:i32)
          n232 = Divide(x=w607, y=w606) -> (x/y=w605:dbl)
          n233 = Array Size(array=w609) -> (size(s)=w610:i32)
          n234 = Add Array Elements(numeric array=w616) -> (sum=w615:dbl)
          n235 = Add Array Elements(numeric array=w609) -> (sum=w611:dbl)
          n236 = Divide(x=w615, y=w614) -> (x/y=w612:dbl)
          n237 = Divide(x=w611, y=w610) -> (x/y=w608:dbl)
        }
        "临界途径平均值" <- w398
        "表象周期平均（秒）" <- w400
        "通量平均值" <- w401
        "选段斜率" <- w399
        n238 = To Double Precision Float(number=w379) -> (double precision float=w378:dbl[])
        n239 = for {
          N -> [w553]
          tunnel: w401 -> [w560] mode=indexing
          tunnel: w400 -> [w552] mode=indexing
          tunnel: w399 -> [w561] mode=indexing
          tunnel: w398 -> [w551] mode=indexing
          shift-right: [w557] -> w388
          shift-left: dbl[] [] -> [w559]
          shift-right: [w554] -> w391
          shift-left: string[] [] ("行首字符串[]") -> [w556]
          tunnel: [w553] -> w383
          n240 = Build Array(w561, w560, w552, w551) -> (w558:dbl[])
          n241 = Insert Into Array(array=w556, new element=string[] ["选段斜率", "通量平均值", "周期平均值", "临界途径值"] ("行首字符串[]")) -> (w554:string[])  [unwired: 1 in]
          n242 = Insert Into Array(array=w559, new element=w558) -> (w557:dbl[])  [unwired: 1 in]
        }
        n243 = Insert Into Array(array=w388, new element=w378) -> (w387:dbl[])  [unwired: 1 in]
        n244 = case shown="False" "添加记录" {
          tunnel: w396 -> [w526 w550]
          tunnel: w387 -> [_ w549]
          tunnel: [w525 w548] -> w386
          tunnel: [w524 TRUE] -> w394
          frame False {
            n245 = property on="Table" class="Tbl (strict)"() -> ("Selection Start"=w533:T6, "Selection Size"=w532:T6)  [unwired: 2 in, 2 out]
            n246 = Unbundle By Name(w533) -> ("Row"=w523:i32)
            n247 = Unbundle By Name(w532) -> ("Row"=w530:i32, "Column"=w520:i32)
            n248 = Equal?(x=1, y=w530) -> (x = y?=w522:bool)
            n249 = Greater Or Equal?(x=w520, y=4) -> (x >= y?=w521:bool)
            n250 = And(x=w522, y=w521) -> (x .and. y?=w528:bool)
            n251 = case shown="True" w528 {
              tunnel: "是否删除该行记录？" ("消息") -> [_ w541]
              tunnel: w523 -> [_ w539]
              tunnel: w526 -> [w535 w538]
              tunnel: [w535 w537] -> w525
              tunnel: [FALSE TRUE] -> w524
              frame False {
              }
              frame True {
                n252 = Two Button Dialog(message=w541) -> (T button?=w540:bool)  [unwired: 2 in]
                n253 = case shown="True" w540 {
                  tunnel: w539 -> [_ w546]
                  tunnel: w538 -> [w542 w545]
                  tunnel: [w542 w543] -> w537
                  frame False {
                  }
                  frame True {
                    n254 = Delete From Array(array=w545, length=1 ("长度"), index (row)=w546) -> (array with subset deleted=w543:dbl[][])  [unwired: 1 in, 1 out]
                  }
                }
              }
            }
          }
          frame True {
            n255 = Insert Into Array(array=w550, new element=w549) -> (w548:dbl[][])  [unwired: 2 in]
          }
        }
        n256 = Multiply(x=w383, y=4) -> (x*y=w381:i32)
        n257 = Delete From Array(array=w386, length=2 ("长度"), index (col)=w381) -> (deleted portion=w377:dbl[][], array with subset deleted=w385:dbl[][])  [unwired: 1 in]
        n258 = Array To Spreadsheet String(array=w385, 3:"%#g" ("格式字符串")) -> (spreadsheet string=w390:string)  [unwired: 1 in]
        n259 = case shown="True" "保存表格" {
          tunnel: w391 -> [_ w503]
          tunnel: w390 -> [_ w501]
          frame False {
          }
          frame True {
            n260 = Array To Spreadsheet String(array=w503, 3:"%s" ("格式字符串")) -> (spreadsheet string=w502:string)  [unwired: 1 in]
            n261 = File Dialog ("文件对话框")(6:"*.txt" ("类型（所有文件）"), 7:"请指定保存路径" ("提示"), 9:"校验.txt" ("默认名称")) -> (0:w494:errorcluster, 1:w495:bool, 3:w496:path)  [unwired: 1 in, 4 out]
            n262 = Concatenate Strings(w502, w501) -> (w500:string)
            n263 = case shown="False" w495 {
              tunnel: w500 -> [w506 _]
              tunnel: w496 -> [w505 _]
              frame False {
                n264 = Open/Create/Replace File(file path (use dialog)=w505, operation (0:open)=T5."replace or create") -> (refnum out=w509:refnum<file>, error out=w511:errorcluster)  [unwired: 4 in, 1 out]
                n265 = Write to Text File(file (use dialog)=w509, text=w506, error in=w511) -> (refnum out=w508:refnum<file>, error out=w507:errorcluster)  [unwired: 1 in, 1 out]
                n266 = Close File(refnum=w508, error in=w507) -> ()  [unwired: 2 out]
              }
              frame True {
              }
            }
            n267 = call <vilib>:"Clear Errors.vi"("error in (no error)"=w494) -> ()  [unwired: 5 in, 2 out]
          }
        }
        n268 = event shown="[0] \"Table\": Mouse Down" {
          selector: _ -> [_ _]
          dyn-events: _ -> [_ _]
          timeout: 20 -> [_ _]
          tunnel: w377 -> [w481 _]
          event "Table": Mouse Down {
            n269 = event-data() -> ("Mods"=w488:cluster{"Double Click":bool, "Menu Key":bool})  [unwired: 1 in]
            n270 = property on="Table" class="Tbl (strict)"() -> ("EditPos"=w486:T6)  [unwired: 2 in, 2 out]
            n271 = Unbundle By Name(w488) -> ("Double Click"=w484:bool)
            n272 = Unbundle By Name(w486) -> ("Row"=w480:i32)
            n273 = Greater Or Equal?(x=w480, y=0) -> (x >= y?=w485:bool)
            n274 = Index Array(array=w481, index (row)=w480) -> (element=w482:dbl[])  [unwired: 1 in]
            n275 = And(x=w484, y=w485) -> (x .and. y?=w483:bool)
            n276 = case shown="True" w483 {
              tunnel: w482 -> [_ w490]
              frame False {
              }
              frame True {
                n277 = To Long Integer(number=w490) -> (32bit integer=w489:i32[])
                n278 = for {
                  tunnel: w489 -> [w491] mode=indexing
                  i -> [w492]
                  n279 = property on="【文件波形】" class="WFGraph (strict)"("Active Cursor"=w492) -> (error out=w493:errorcluster)  [unwired: 2 in, 1 out]
                  n280 = property on="【文件波形】" class="WFGraph (strict)"(error in=w493, "Cursor.Cursor Index"=w491) -> ()  [unwired: 1 in, 2 out]
                }
              }
            }
          }
          event Timeout {
            n281 = event-data() -> ()  [unwired: 1 in, 1 out]
          }
        }
        n282 = case shown="True" w394 {
          tunnel: w391 -> [_ w513]
          tunnel: w390 -> [_ w512]
          frame False {
          }
          frame True {
            n283 = property on="Table" class="Tbl (strict)"("Column Headers[]"=w513, "Col Headers Vis"=TRUE ("显示项:显示列首")) -> (error out=w515:errorcluster)  [unwired: 2 in, 1 out]
            n284 = Spreadsheet String To Array(format string="%s" ("格式字符串"), spreadsheet string=w512, array type (2D Dbl)=string[][] [] ("添加的数组")) -> (array=→"Table":string[][])  [unwired: 1 in]
            n285 = property on="Table" class="Tbl (strict)"(error in=w515, "Selection Size"=T6 {"Row"=0, "Column"=0} ("选择区域大小")) -> ()  [unwired: 1 in, 2 out]
          }
        }
        n286 = local read "退出程序"() -> (w415:bool)
      }
    }
    frame #3 {
      n287 = invoke class="VI" method="FP.Close"() -> (reference out=w619:refnum<vi>, error out=w618:errorcluster)  [unwired: 3 in, 1 out]
      n288 = Close Reference(reference=w619, error in (no error)=w618) -> ()  [unwired: 1 out]
    }
  }
